vi "Weighting Filter.vi"(4 "weighting filter init/cont (init:F)":bool, 5 "type":enum16{"Type 0", "Type 1"}(ring)=enum."Type 1", 6 "channel info IN":T1={"sensor sensitivity [mV/EU]"=1000.0, "engineering units"=1, "dB reference [EU]"=1.0, "custom label"="EU", "weighting filter"=0, "pregain [dB]"=0.0} {"pregain [dB]" format="%.2f"; "weighting filter" items=["Linear", "A-weighting", "B-weighting", "C-weighting", "ITU-R 468-4", "Dolby", "CCITT", "C-message"]; "dB reference [EU]" format="%^.1e"; "engineering units" items=["custom..."=0, "V"=1, "A"=21, "Pa"=2, "N"=20, "g"=3, "m/s^2"=4, "m/s"=5, "m"=6, "mm/s"=12, "mm"=13, "microns/s"=14, "microns"=15, "in/s^2"=7, "in/s"=8, "in"=9, "mils/s"=10, "mils"=11, "rad/s^2"=16, "rad/s"=17, "rad"=18, "strain"=19]; "sensor sensitivity [mV/EU]" format="%.2f"}, 7 "weighting filter":T4(ring)=enum."A-weighting", 8 "sampling frequency [Hz]":dbl=10000.0 format="%.2f", 9 "scaled signal [EU]":dbl[](array[numeric]) format="%.2f") -> (0 "channel info OUT":T1={"sensor sensitivity [mV/EU]"=1000.0, "engineering units"=1, "dB reference [EU]"=1.0, "custom label"="EU", "weighting filter"=0, "pregain [dB]"=0.0} {"pregain [dB]" format="%.2f"; "weighting filter" items=["Linear", "A-weighting", "B-weighting", "C-weighting", "ITU-R 468-4", "Dolby", "CCITT", "C-message"]; "dB reference [EU]" format="%^.1e"; "engineering units" items=["custom..."=0, "V"=1, "A"=21, "Pa"=2, "N"=20, "g"=3, "m/s^2"=4, "m/s"=5, "m"=6, "mm/s"=12, "mm"=13, "microns/s"=14, "microns"=15, "in/s^2"=7, "in/s"=8, "in"=9, "mils/s"=10, "mils"=11, "rad/s^2"=16, "rad/s"=17, "rad"=18, "strain"=19]; "sensor sensitivity [mV/EU]" format="%.2f"}, 1 "weighting conflict":bool, 2 "max freq within tolerances [Hz]":dbl format="%.2f", 3 "weighted signal [EU]":dbl[](array[numeric]) format="%.2f")   [LabVIEW 2017]
doc: "Applies the selected weighting filter (A, B, or C) on the input signal.\nBased on the selected type (Type 1 or Type 0), this VI returns the maximum frequency within tolerances for this particular type.\nTo ensure continuous filtering operation, call this VI the first time with weighting filter init/cont set to FALSE and then call it with weighting filter init/cont set to TRUE."
uses:
  <vilib>/addons/Sound and Vibration/compatibility/Controls/svl_Channel Info.ctl
  <vilib>/addons/Sound and Vibration/compatibility/Controls/svl_Engineering Units Text Ring.ctl
  <vilib>/addons/Sound and Vibration/compatibility/Controls/svl_Weighting Filter Text Ring.ctl
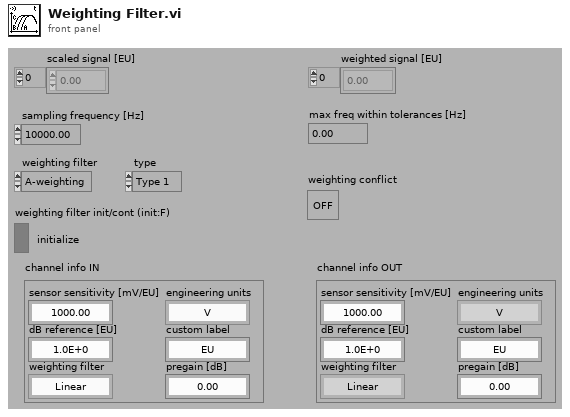
[diagram p1: front panel]
types:
  T1 = typedef "svl_Channel Info.ctl" = cluster{"sensor sensitivity [mV/EU]":dbl, "engineering units":T2, "dB reference [EU]":dbl, "custom label":string, "weighting filter":T3, "pregain [dB]":dbl}
  T2 = typedef "svl_Engineering Units Text Ring.ctl" = u16
  T3 = typedef "svl_Weighting Filter Text Ring.ctl" = u16
  T4 = enum16{"Linear", "A-weighting", "B-weighting", "C-weighting"}
  T5 = cluster{"filter structure":enum32{"IIR 2nd Order", "IIR 4th Order"}, "Reverse Coefficients":dbl[], "Forward Coefficients":dbl[]}
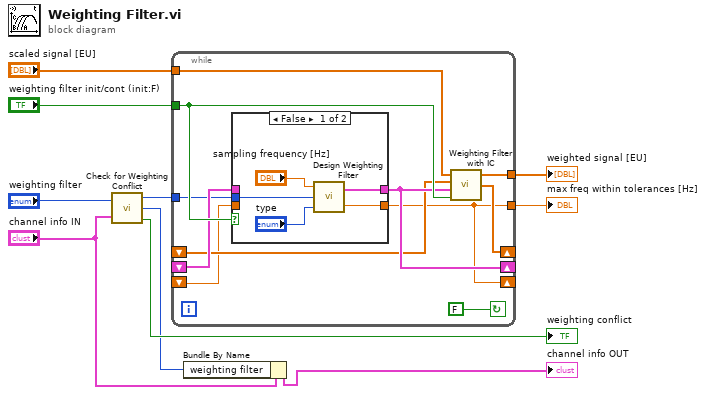
[diagram p0: block diagram]
diagram:
  n1 = call <vilib>:"Check for Weighting Conflict.vi"("weighting filter"="weighting filter", "channel info"="channel info IN") -> ("weighting to apply"=w6:T4, "weighting units"=w1:T4, "weighting conflict"=→"weighting conflict":bool)
  n2 = while {
    shift-left: _ -> [w12]
    shift-right: [w13] -> _
    tunnel: [w13] -> w3
    tunnel: w6 -> [w14]
    shift-left: _ -> [w18]
    shift-right: [w17] -> _
    tunnel: [w19] -> w8
    shift-left: _ -> [w16]
    shift-right: [w15] -> _
    tunnel: "scaled signal [EU]" -> [w20]
    tunnel: "weighting filter init/cont (init:F)" -> [w21]
    stop <- FALSE continue-if-true
    n3 = case shown="False" w21 {
      tunnel: [w25 w28] -> w17
      tunnel: w18 -> [_ w28]
      tunnel: w14 -> [w24 _]
      tunnel: [w22 w27] -> w13
      tunnel: w12 -> [_ w27]
      frame False {
        n4 = call <vilib>:"Design Weighting Filter.vi"("type"="type", "weighting"=w24, "sampling frequency [Hz]"="sampling frequency [Hz]") -> ("max freq within tolerances [Hz]"=w22:dbl, "filter coefficients"=w25:T5)
      }
      frame True {
      }
    }
    n5 = call <vilib>:"Weighting Filter with IC.vi"("init/cont (init:F)"=w21, "filter coefficients"=w17, "initial filter state"=w16, "X"=w20) -> ("final filter state"=w15:dbl[], "filtered X"=w19:dbl[])  [unwired: 1 out]
  }
  "weighted signal [EU]" <- w8
  "max freq within tolerances [Hz]" <- w3
  n6 = Bundle By Name(cluster="channel info IN", "weighting filter"=w1) -> (→"channel info OUT":T1)
